vi "adjustable_lookup_for_image_display (SubVI).vi"(9 "Mid-level value":u16, 10 "Minimum value":u16, 11 "Maximum value":u16) -> (3 "User-defined Look-up table":u16[](array[numeric]))   [LabVIEW 2016]
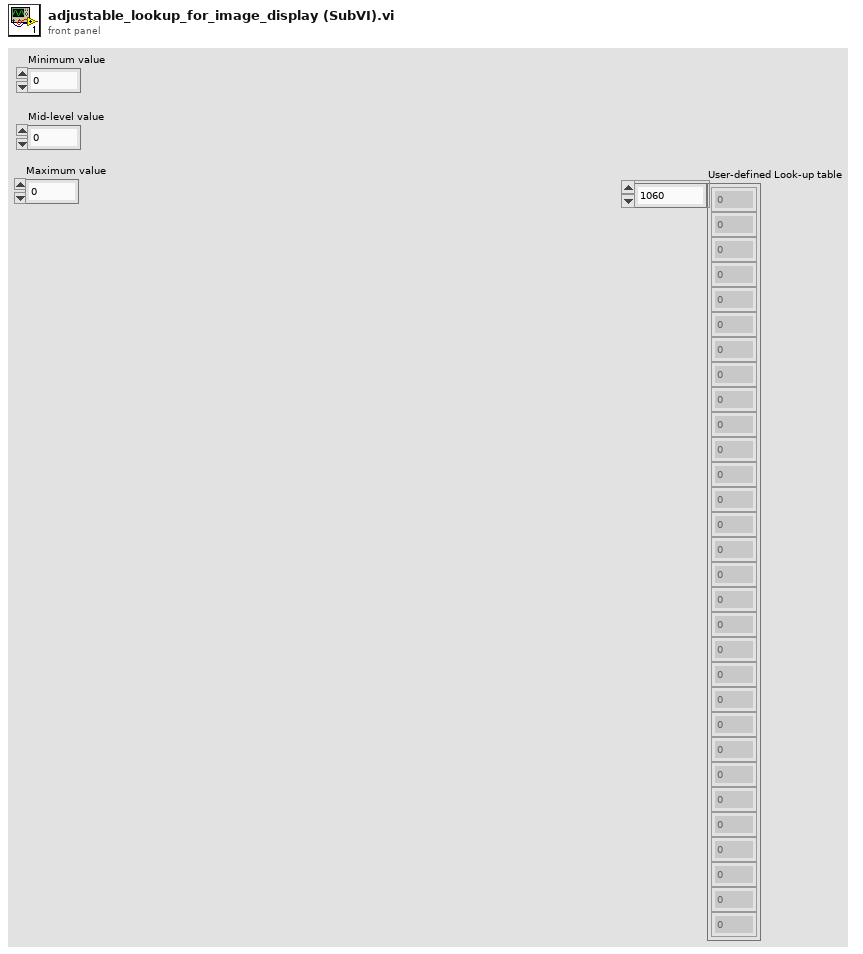
[diagram p1: front panel]
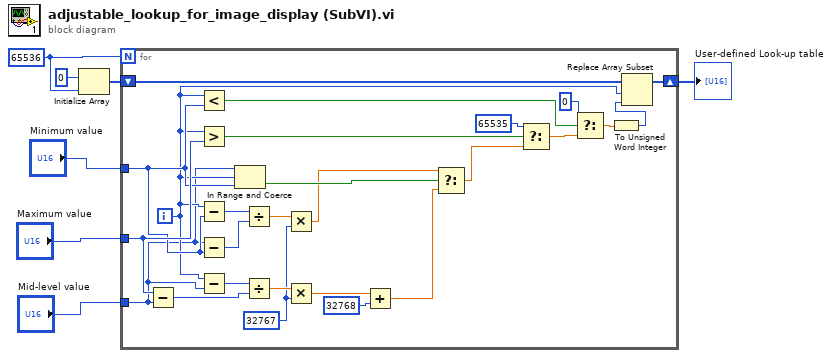
[diagram p0: block diagram]
diagram:
  w1 = 65536 ("dimension size")
  n1 = Initialize Array(u16 0 ("element"), w1) -> (w2:u16[])
  n2 = for {
    N: w1 -> [_]
    shift-right: [w32] -> w6
    shift-left: w2 -> [w33]
    tunnel: "Minimum value" -> [w10]
    tunnel: "Maximum value" -> [w23]
    tunnel: "Mid-level value" -> [w8]
    i -> [w9]
    w17 = u16 32767 ("y")
    n3 = Subtract(x=w23, y=w8) -> (x-y=w22:u16)
    n4 = Less?(x=w9, y=w10) -> (x < y?=w30:bool)
    n5 = Greater?(x=w9, y=w23) -> (0:w28:bool)
    n6 = Subtract(x=w9, y=w10) -> (x-y=w21:i32)
    n7 = Subtract(x=w8, y=w10) -> (x-y=w20:u16)
    n8 = Subtract(x=w9, y=w8) -> (x-y=w19:i32)
    n9 = In Range and Coerce(upper limit=w8, x=w9, lower limit=w10) -> (In Range?=w24:bool)  [unwired: 1 out]
    n10 = Divide(x=w21, y=w20) -> (x/y=w26:dbl)
    n11 = Divide(x=w19, y=w22) -> (x/y=w18:dbl)
    n12 = Multiply(x=w26, y=w17) -> (x*y=w14:dbl)
    n13 = Multiply(x=w18, y=w17) -> (x*y=w16:dbl)
    n14 = Add(x=w16, y=u16 32768) -> (x+y=w13:dbl)
    n15 = Select(t=w14, s=w24, f=w13) -> (s? t:f=w25:dbl)
    n16 = Select(t=u16 65535, s=w28, f=w25) -> (s? t:f=w29:dbl)
    n17 = Select(t=u16 0, s=w30, f=w29) -> (s? t:f=w11:dbl)
    n18 = To Unsigned Word Integer(number=w11) -> (unsigned 16bit integer=w12:u16)
    n19 = Replace Array Subset(array=w33, new element=w12, index=w9) -> (w32:u16[])
  }
  "User-defined Look-up table" <- w6
